vi "FocalMain.vi"() -> ()   [LabVIEW 2018]
uses:
  Clusters/FileDataChannel.ctl
  Clusters/WindSimMode.ctl
  Clusters/SimulationConstants.ctl
  Clusters/BladePitchMode.ctl
  Clusters/GenMode.ctl
  <vilib>/Platform/TimedLoop/XDataNode/timing_clust.ctl
  <vilib>/Platform/TimedLoop/XDataNode/nitl_modes.ctl
  <vilib>/Platform/TimedLoop/XDataNode/wakeup.ctl
  Clusters/IOSignals.ctl
  Clusters/RoscoParams.ctl
  Clusters/ArrayPairs.ctl
  Clusters/SwapArrayCluster.ctl
  Clusters/PitchCtrl.ctl
  Clusters/GenCtrl.ctl
  Clusters/ScalingEnum.ctl
  <vilib>/Utility/file.llb/Read Delimited Spreadsheet (DBL).vi
  SubVIs/InsertIntoArray_v2.vi
  <vilib>/platform/TimedLoop/XDataNode/XDataNode.xnode
  <vilib>/Platform/TimedLoop/XDataNode/XDNodeRunTimeDep.lvlib
  <resource>/objmgr/IndComECAT.rc
  <vilib>/ptbypt/NI_PtbyPt.lvlib
panel:
  out "error out":errorcluster
  in  "Torque Ctrl P-Gain":dbl=1.0
  in  "Pitch I-Gain":dbl
  out "Torque RAW (V)":dbl
  in  "Max Torque (MNm)":dbl=20.0
  in  "Velocity Ctrl I-Gain":dbl=0.5
  in  "Velocity Ctrl P-Gain":dbl=0.1
  in  "Torque Ctrl I-Gain":dbl=1.0
  out "Torque sine period MS (Nm) 2":dbl
  out "Torque sine amp MS (Nm)":dbl
  out "Torque setpoint (Nm)":dbl
  out "Torque Sensor (Nm)":dbl(knob) scale=-2.0..2.0
  in  "Torque sine period (s)":dbl=100.0
  in  "Torque sine amp (MNm)":dbl
  out "Motor Torque (Nm)":dbl(knob) scale=-2.0..2.0
  out "Torque sine mean MS (Nm)":dbl
  in  "Torque mean (MNm)":dbl
  out "Ramp time MS (s)":dbl
  out "Ramp target vel MS (rpm)":dbl
  out "Const. vel setpoint MS (rpm)":dbl
  in  "Ramp time (s)":dbl=100.0
  in  "Ramp target vel (rpm)":dbl=10.0
  in  "Const. vel setpoint (rpm)":dbl
  out "Sine period MS (s)":dbl
  out "Sine amp MS (deg)":dbl
  out "Sine Mean MS (deg)":dbl
  out "Const. setpoint MS (deg)":dbl
  in  "Generator operating mode":T1
  in  "Sine period (s)":dbl=100.0
  in  "Sine amp (deg)":dbl=15.0
  in  "Sine mean (deg)":dbl=1.0
  in  "Const. setpoint (deg)":dbl=10.0
  in  "Blade pitch operating mode":T2
  out "SIM-GenTorque_Nm":dbl
  in  "Wind Est. u(t=0)":dbl=5.0
  out "Wind Speed (m/s)":dbl
  out "Ramp time (s)":dbl
  in  "Ramp Time (s)":dbl=500.0
  in  "Ramp End u(m/s)":dbl=15.0
  in  "Ramp Start u(m/s)":dbl=5.0
  in  "Const. Amp (m/s)":dbl=5.0
  in  "Wind Simulation Mode":T3
  out "File Write (s)":dbl format="%5.1f"
  out "File Name":string
  out "State logic late?":bool
  out "Actual shaft Speed MS (rpm)":dbl(knob)=7.068579725455493e-05 scale=-100.0..100.0
  in  "Pitch P-Gain":dbl=12.0
  out "Axis 3 Fault":bool
  out "Axis 3 Warning":bool
  out "Axis 2 Fault":bool
  out "Axis 2 Warning":bool
  out "Axis 1 Fault":bool
  out "Axis 1 Warning":bool
  out "Axis 3 Operational":bool
  out "Axis 2 Operational":bool
  out "Axis 1 Operational":bool
  out "Pitch Axis 3":string
  out "Pitch Axis 2":string
  out "Pitch Axis 1":string
  in  "Clear Pitch Actuator Faults (x3)":bool
  in  "Enable Pitch Actuators (x3)":bool
  out "MS Pitch Blade 3 (deg)":dbl(knob) scale=0.0..30.0 scale format="%.2f"
  out "MS Pitch Blade 2 (deg)":dbl(knob) scale=0.0..30.0 scale format="%.2f"
  out "MS Pitch Blade 1 (deg)":dbl(knob) scale=0.0..30.0 scale format="%.2f"
  out "Generator Operational":bool
  in  "Clear Accelnet Faults":bool
  in  "Enable Accelnet":bool
  out "Generator Fault":bool
  out "Generator Warning":bool
  out "Main generator state":string
  out "Rosco Failed?":bool
  in  "Sine Freq (Hz)":dbl=0.009999999776482582
  in  "Sine Mean (m/s)":dbl=7.0
  in  "Sine Amp (m/s)":dbl
  out "Generator Torque (MNm)":dbl(knob) scale=0.0..35.0
  out "Generator Speed (rpm)":dbl(knob)=7.068579725455493e-05 scale=0.0..10.0
  in  "?":T4(tab)
  out "Generator Speed (ROSCO / SIM)":dynamicdata(graph)
  out "Torque (ROSCO/ SIM)":dynamicdata(graph)
  out "Pitch MS (ROSCO)":dynamicdata(graph)
  out "TSR":dynamicdata(graph)
  out "Generator Speed MS (Manual)":dynamicdata(graph)
  out "Pitch MS (Manual)":dynamicdata(graph)
  out "Torque MS (Manual)":dynamicdata(graph)
  out "Aero Torque":dynamicdata(graph)
  out "WindSpeed(m/s)":dbl(graph)
  in  "To VS_ControlMode":T5(ring)
  in  "Edit DISCON":bool
  out "DISCON.IN Contents":string
  in  "From VS_ControlMode":T5(ring)
  out "Rosco Return Message":string
  out "Setpoints":dbl[][](array[numeric])
  out "Pitch FS (deg)":dbl
  out "Time index":i32
  out "Time FS (s)":dbl
  out "Vel FS (rpm)":dbl
  out "Loop duration (ms)":i64
  out "Pitch axis 3 ctrl word":u16 format="%x"
  out "Pitch axis 2 ctrl word":u16 format="%x"
  out "avrSWAP":sgl[](array[numeric])
  out "OUT_DEBUG":dbl
  out "RT Loop Duration":i64
  out "Control Mode - Main Gen":u8
  out "WriteSDO Abort - Main Gen":u32
  out "ReadSDO Abort - Main Gen":u32
  out "Gen ctrl word":u16 format="%x"
  out "Pitch axis 1 ctrl word":u16 format="%x"
  out "Graphics Update t (s)":dbl format="%.1f"
  out "Effective rate (ms)":dbl format="%#.1f"
  out "WriteSDO Abort - Pitch 1":u32
  out "ReadSDO Abort - Pitch 1":u32
  out "Control Mode - Pitch 1":u8
  in  "Zero Pitch 1":bool
  in  "Zero Pitch 2":bool
  in  "Zero Pitch 3":bool
  out "SIM-Cp":dbl
  out "OUT_AEROTQ":dbl
  out "OUT_ROTSP":dbl
  out "SimulationConst":T6={"Ngear"=1.0, "RotorInertia"=318628128.0, "GeneratorEff"=0.9700000286102295, "RotorRadius"=120.0, "Rho"=1.225000023841858, "NumBlades"=1, "ScaleFactor"=3.0} {"RotorInertia" format="%.2f"}
  out "Scan Engine Mode":i32(ring)=2 items=["Initialization Mode", "Configuration Mode", "Active Mode", "Fault Mode"]
  out "Torque Setpoint (MNm)":dbl(knob) scale=0.0..35.0
  out "Pitch Setpoint (deg)":dbl(knob) scale=0.0..30.0 scale format="%.2f"
  out "Power (MW)":dbl(slide) scale=0.0..25.0 scale format="%.2f"
  out "SimLoop Late?":bool
  out "FIFO Loop Late?":bool
  in  "Base filename":string="rosco-tests"
  out "Writing":bool
  in  "WriteData":bool
  in  "?":T7
  out "#RT FIFO":u32
  in  "Stop LabVIEW":bool
  out "Time(s)":dbl format="%6.1f"
  out "RT Loop Late?":bool
  # "FOCAL Campaign 1"
  # "Processed quantities"
  # "FILEWRITING"
  # "MAIN GEN CONTROL"
  # "GENERATOR SIGNALS"
  # "PITCH ACTUATORS CONTROL"
  # "BLADE PITCH SIGNALS"
  # "ROSCO"
  # "WIND SPEED SIMULATOR"
  # "Axis 1"
  # "Axis 2"
  # "Axis 3"
  # "Operational"
  # "Warning"
  # "Error"
  # "Enter FS values"
  # "MS values"
  # "Enter FS values"
  # "MS values"
  # "TURBINE SPECIFICATIONS"
  # "RATED POWER: 15000000 W"
  # "RATED TORQUE: 19624046.66 Nm"
  # "RATED GEN SPEED: 0.79168 rad/s"
  # "ROSCO INPUTS"
  # "Pitch (deg)"
  # "Fan 1"
  # "Fan 20"
  # "Time"
  # "Vel (rpm)"
  # "Fan 10"
  # "Fan 30"
  # "SYSTEM"
  # "ROSCO"
  # "MAIN MOTOR"
  # "PITCH AXIS 1"
  # "PITCH AXIS 2"
  # "PITCH AXIS 3"
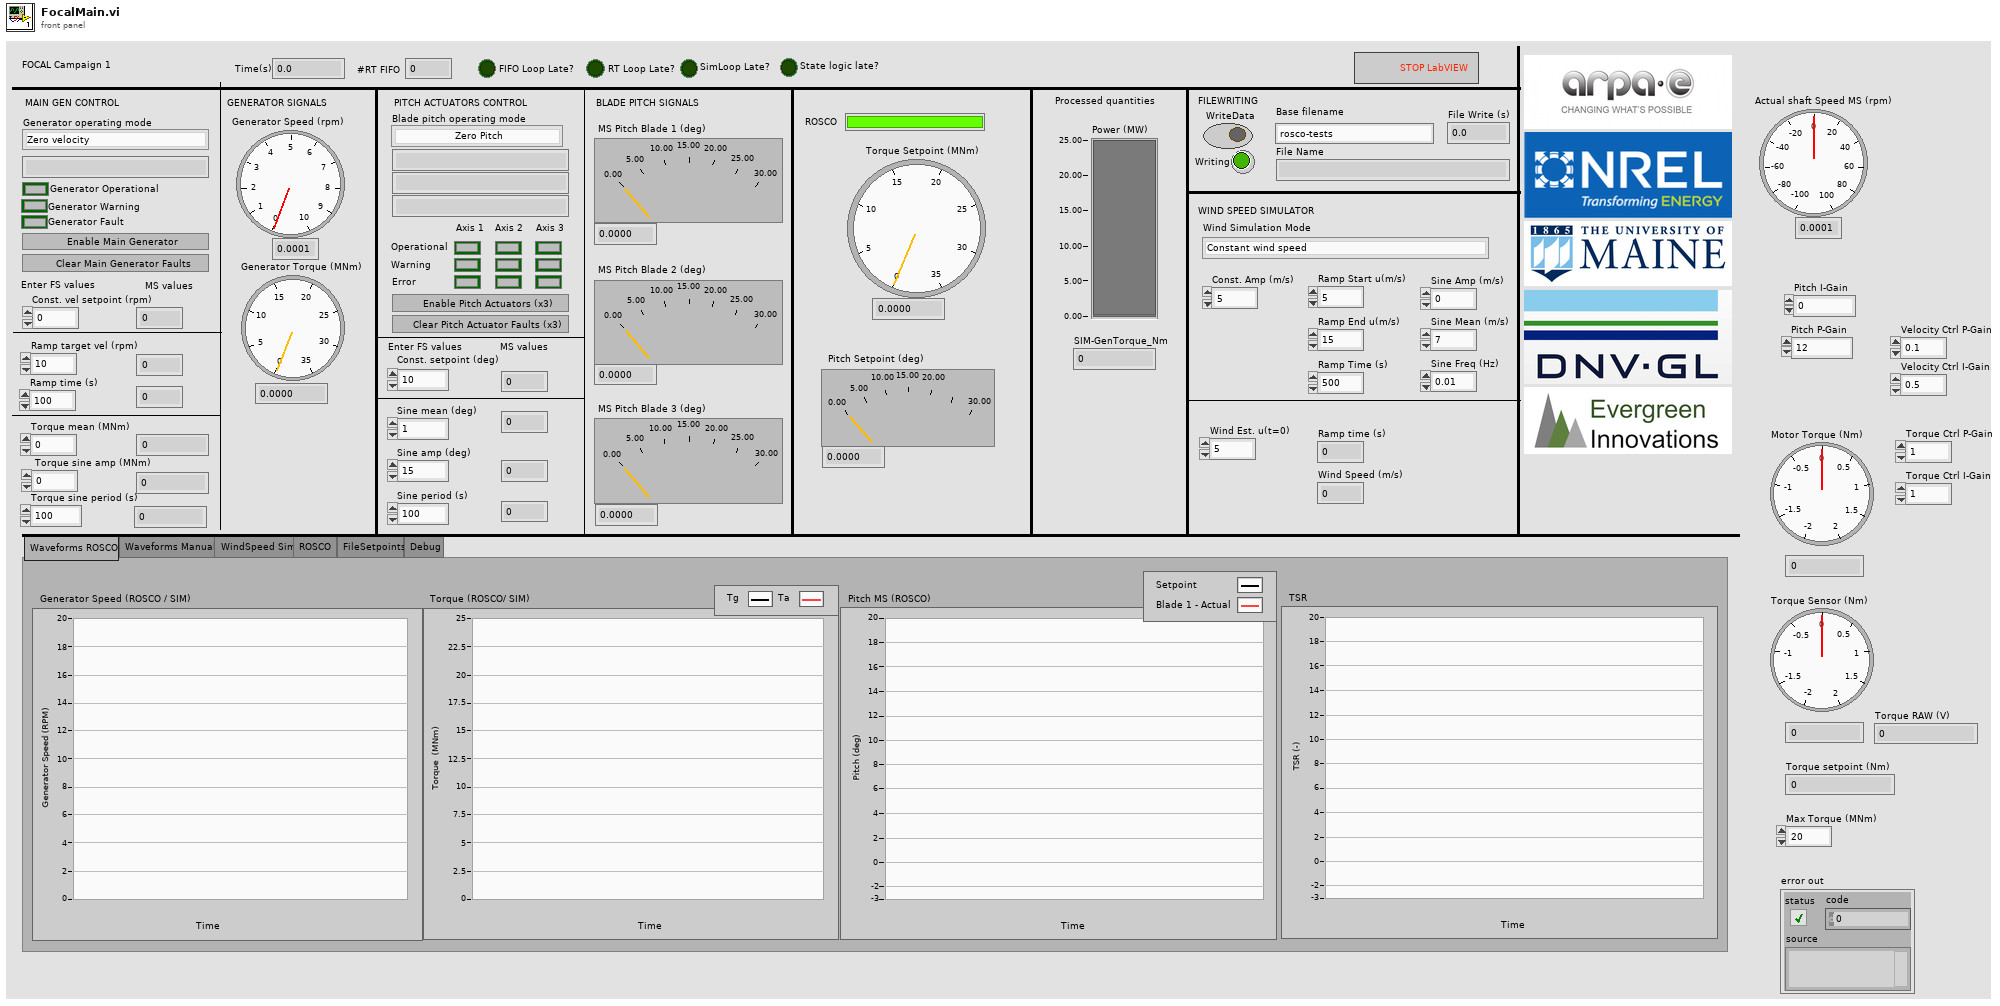
[diagram p1: front panel]
types:
  T1 = typedef "GenMode.ctl" = enum16{"Zero velocity", "Velocity from File", "Constant velocity", "Ramped Velocity", "Sine Torque", "ROSCO"}
  T2 = typedef "BladePitchMode.ctl" = enum16{"Zero Pitch", "Pitch from File", "Constant pitch angle", "Harmonic pitch angle", "ROSCO controlled"}
  T3 = typedef "WindSimMode.ctl" = enum16{"Constant wind speed", "Ramped wind speed", "Sine wind speed"}
  T4 = enum32{"Waveforms ROSCO", "Waveforms Manual", "WindSpeed Sim", "ROSCO", "FileSetpoints", "Debug"}
  T5 = enum16{"Constant Torque", "Constant Power", "PI Control"}
  T6 = typedef "SimulationConstants.ctl" = cluster{"Ngear":dbl, "RotorInertia":dbl, "GeneratorEff":dbl, "RotorRadius":sgl, "Rho":dbl, "NumBlades":i32, "ScaleFactor":dbl}
  T7 = typedef "FileDataChannel.ctl" = cluster{"genSpeed_rad_s":dbl, "genTorque_Nm":dbl, "dataLoopCounter":dbl, "genStatus":dbl, "pitch1Position_rad":dbl, "pitch1Velocity_rad_s":dbl, "pitch1Status":dbl, "dataTime_s":dbl, "genPosition_rad":dbl, "pitch2Position_rad":dbl, "pitch2Velocity_rad_s":dbl, "pitch2Status":dbl, "pitch3Position_rad":dbl, "pitch3Velocity_rad_s":dbl, "pitch3Status":dbl, "pitchSetpoint_rad":dbl, "torqueSetpoint_Nm":dbl, "simUWind_m_s":dbl, "simGenSpeed_rad_s":dbl, "simTa_Nm":dbl, "simCp":dbl}
  T8 = typedef "IOSignals.ctl" = cluster{"mainGenPosition (rad)":dbl, "mainGenTorque (Nm)":dbl, "mainGenVelocity (rad/s)":dbl, "mainGenStatus":u16, "pitch1Position (rad)":dbl, "pitch1Velocity (rad/s)":dbl, "pitch1Status":u16, "pitch2Position (rad)":dbl, "pitch2Velocity (rad/s)":dbl, "pitch2Status":u16, "pitch3Position (rad)":dbl, "pitch3Velocity (rad/s)":dbl, "pitch3Status":u16, "pitch1PosOfst (rad)":dbl, "pitch2PosOfst (rad)":dbl, "pitch3PosOfst (rad)":dbl, "torqueSensor (Nm)":dbl}
  T9 = typedef "RoscoParams.ctl" = cluster{"avrSWAP":sgl[], "aviFAIL":i32, "avcMSG":string, "ReturnValue":i32}
  T10 = typedef "ArrayPairs.ctl" = cluster{"iStatus":T11, "TIME":T11, "DT":T11, "Blade1PitchPos_rad":T11, "VS_MECHGENPWR":T11, "VS_GENPWR":T11, "GEN_SPEED":T11, "ROTOR_SPEED":T11, "GENTQMEAS":T11, "Y_M":T11, "HORWINDV":T11, "ROOTMOOP1":T11, "ROOTMOOP2":T11, "Blade2PitchPos_rad":T11, "Blade3PitchPos_rad":T11, "ROOTMOOP3":T11, "AVCMSG_SIZE":T11, "INFILE_SIZE ":T11, "OUTFILE_SIZE ":T11, "FA_ACC":T11, "NUM_BLADES":T11, "BladePitchSetpoint_rad":T11, "TorqueSetpoint_Nm":T11, "OUT_AEROTQ":T11, "Out.RotSpeed ":T11, "Out.DEBUG":T11}
  T11 = typedef "SwapArrayCluster.ctl" = cluster{"Index":i32, "Value":dbl}
  T12 = typedef "XDNodeRunTimeDep.lvlib/timing_clust.ctl" = cluster{"Expected End [f-1]":u64, "Actual End [f-1]":u64, "Finished Late? [f-1]":bool, "Expected End [i-1]":u64, "Actual End [i-1]":u64, "Finished Late? [i-1]":bool, "Expected Start [i]":u64, "Actual Start [i]":u64, "Expected Start [f]":u64, "Actual Start [f]":u64, "Source Name":string, "Structure Name":string, "Period":i64, "Deadline":i64, "Offset":i64, "Start":i64, "Priority":i32, "Timeout":i32, "Mode":T13, "Wakeup Reason":T14, "Error":errorcluster, "Source Type":string, "Secondary Source Type":string, "Global End Time":u64, "Global Start Time":u64, "Frame Duration":u64, "Iteration Duration":u64, "Assigned CPU":i32, "I/O Scan Engine Mode":u32}
  T13 = typedef "XDNodeRunTimeDep.lvlib/nitl_modes.ctl" = enum32{"No Change", "Process missed periods, maintain original phase", "Discard missed periods, maintain original phase", "Process missed periods, ignore original phase", "Discard missed periods, ignore original phase"}
  T14 = typedef "XDNodeRunTimeDep.lvlib/wakeup.ctl" = enum32{"Normal", "Aborted", "Asynchronous wakeup", "Timing source error", "Timed loop error", "Timeout"}
  T15 = typedef "PitchCtrl.ctl" = cluster{"P-Gain":dbl, "Blade pitch operating mode":T2, "Constant setpoint (deg)":dbl, "Sine mean (deg)":dbl, "Sine amp (deg)":dbl, "Sine period (s)":dbl, "I-Gain":dbl, "Axis 1 On":bool, "Axis 2 On":bool, "Axis 3 On":bool, "Pitch from File (deg)":dbl}
  T16 = typedef "GenCtrl.ctl" = cluster{"Generator operating mode":T1, "Constant velocity setpoint (rpm)":dbl, "Ramp target velocity (rpm)":dbl, "Ramp time (s)":dbl, "Sine mean (Nm)":dbl, "Sine amp (Nm)":dbl, "Sine period (s)":dbl, "Torque Ctrl I-Gain":dbl, "Velocity Ctrl P-Gain":dbl, "Velocity Ctrl I-Gain":dbl, "Max Torque (Nm)":dbl, "GeneratorOn":bool, "Torque Ctrl P-Gain":dbl, "From file velocity (rpm)":dbl}
  T17 = typedef "ScalingEnum.ctl" = enum16{"Model scale -> Full scale", "Full scale -> Model scale"}
  T18 = typedef "ElmoState.ctl" = cluster{"Elmo State":string, "Elmo Operational":bool, "Elmo Warning":bool, "Elmo Fault":bool}
  T19 = typedef "AccelnetState.ctl" = cluster{"State String":string, "Accelnet Warning":bool, "Accelnet Fault":bool, "Accelnet Operational":bool}
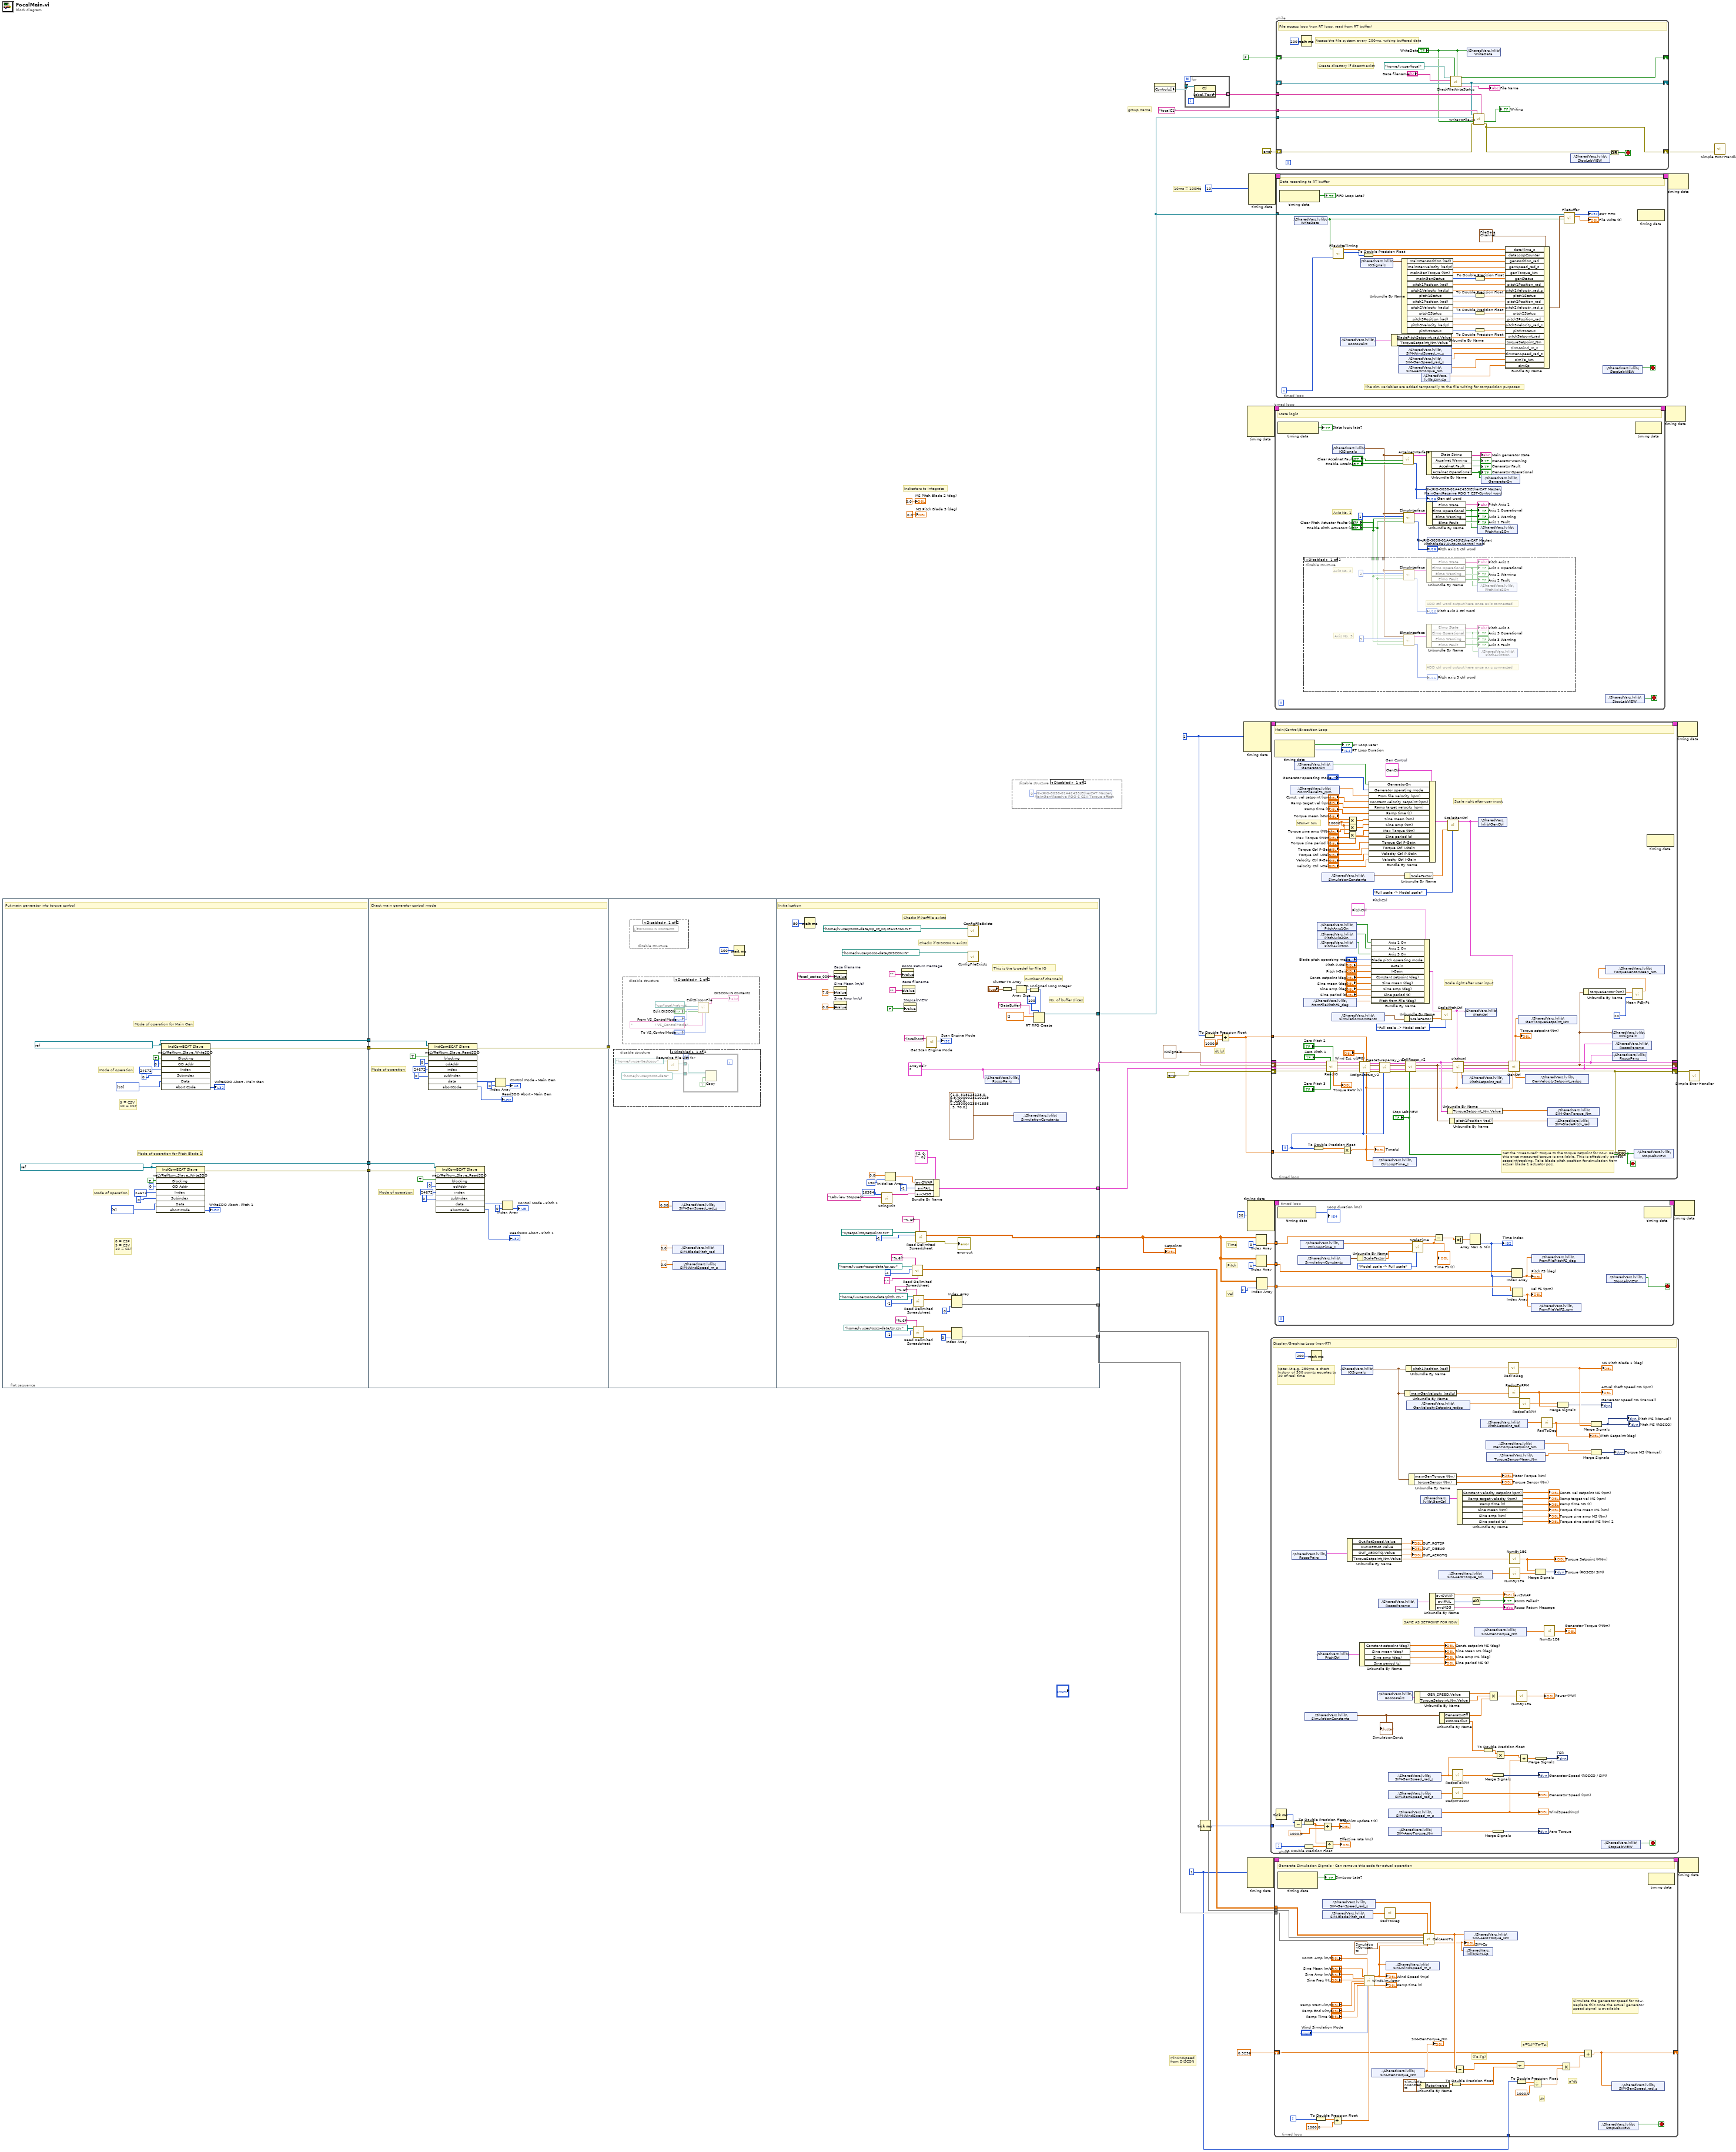
[diagram p0: block diagram]
diagram:
  w16 = i64 2 ("Period")
  w23 = i64 1 ("Period")
  # "Vel"
  # "Pitch"
  # "Time"
  # "MinOMSpeed\nfrom DISCON"
  # "dt (s)"
  # "10ms = 100Hz"
  # "group name"
  # "Indicators to integrate"
  n1 = flat-sequence {
    tunnel: [w57] -> w33
    tunnel: [w58] -> w32
    tunnel: [w50] -> w25
    tunnel: [w49] -> w24
    tunnel: w33 -> [w77]
    tunnel: w32 -> [w76]
    tunnel: [w75] -> w31
    tunnel: w25 -> [w66]
    tunnel: w24 -> [w65]
    tunnel: w31 -> [_]
    tunnel: [w146] -> w27
    tunnel: [w139] -> w40
    tunnel: [w125] -> w39
    tunnel: [w128] -> w38
    tunnel: [w127] -> w37
    tunnel: [w110] -> w36
    tunnel: [w103] -> w4
    frame #0 {
      w50 = refnum<k21> "ni.var.io://ni-crio-9038-01a42455/EtherCAT Master/PitchBlade1" ("Slave Constant")
      w57 = refnum<k21> "ni.var.io://ni-crio-9038-01a42455/EtherCAT Master/MainGen" ("Slave Constant")
      # "Mode of operation for Pitch Blade 1"
      # "Mode of operation for Main Gen"
      # "Mode of operation"
      # "8 = CSP \n9 = CSV\n10 = CST"
      # "Mode of operation"
      # "9 = CSV\n10 = CST"
      # "Put main generator into torque control"
      n2 = invoke class="IndComECAT Slave" method="neLVRefNum_Slave_WriteSDO"(reference=w50, "Blocking"=TRUE, "OD Addr"=u16 0, "Index"=u16 24672, "Subindex"=u8 0, "Data"=u8[] [9]) -> (error out=w49:errorcluster, "Abort Code"=→"WriteSDO Abort - Pitch 1":u32)  [unwired: 3 in, 7 out]
      n3 = invoke class="IndComECAT Slave" method="neLVRefNum_Slave_WriteSDO"(reference=w57, "Blocking"=TRUE, "OD Addr"=u16 0, "Index"=u16 24672, "Subindex"=u8 0, "Data"=u8[] [10]) -> (error out=w58:errorcluster, "Abort Code"=→"WriteSDO Abort - Main Gen":u32)  [unwired: 3 in, 7 out]
    }
    frame #1 {
      # "Mode of operation"
      # "Mode of operation"
      # "Check main generator control mode"
      n4 = invoke class="IndComECAT Slave" method="neLVRefNum_Slave_ReadSDO"(reference=w77, error in=w76, "blocking"=TRUE, "odAddr"=u16 0 ("OD address"), "index"=u16 24672 ("Index"), "subIndex"=u8 0 ("Subindex")) -> (error out=w75:errorcluster, "data"=w80:u8[], "abortCode"=→"ReadSDO Abort - Main Gen":u32)  [unwired: 3 in, 6 out]
      n5 = invoke class="IndComECAT Slave" method="neLVRefNum_Slave_ReadSDO"(reference=w66, error in=w65, "blocking"=TRUE, "odAddr"=u16 0 ("OD address"), "index"=u16 24672 ("Index"), "subIndex"=u8 0 ("Subindex")) -> ("data"=w69:u8[], "abortCode"=→"ReadSDO Abort - Pitch 1":u32)  [unwired: 3 in, 7 out]
      n6 = Index Array(array=w80, index=0) -> (element=→"Control Mode - Main Gen":u8)
      n7 = Index Array(array=w69, index=0) -> (element=→"Control Mode - Pitch 1":u8)
    }
    frame #2 {
      n8 = disable-structure shown="Disabled" {
        frame Disabled {
          n9 = call <vilib>:"Recursive File List.vi"("Folder Path"=path "/home/lvuser/testcopy" ("path")) -> ("All Files in Dir"=w91:path[])  [unwired: 6 in, 4 out]
          n10 = for {
            tunnel: path "/home/lvuser/rosco-data" ("target path (use dialog)") -> [w95]
            tunnel: w91 -> [w94] mode=indexing
            n11 = Copy(9:TRUE ("overwrite (F)"), 10:w95, 11:w94) -> ()  [unwired: 2 in, 3 out]
          }
        }
        frame Enabled {
        }
      }
      n12 = disable-structure shown="Disabled" {
        frame Disabled {
          n13 = call "EditDisconFile.vi"("To VS_ControlMode"="To VS_ControlMode", "Append"="                   ! VS_ControlMode", "Edit DISCON"="Edit DISCON", "From VS_ControlMode"="From VS_ControlMode", "path"=path "/usr/local/natinst/labview/DISCON.IN") -> ("data"=→"DISCON.IN Contents":string)  [unwired: 4 in, 1 out]
        }
        frame Enabled {
        }
      }
      n14 = disable-structure shown="Disabled" {
        frame Disabled {
          n15 = local read "DISCON.IN Contents"() -> ()  [unwired: 1 in]
        }
        frame Enabled {
        }
      }
      n16 = shared-variable ".\\SharedVars.lvlib\\SIM-GenSpeed_rad_s"(0.009999999776482582 ("RotorSpeed(rad/s)")) -> ()  [unwired: 1 in, 1 out]
      n17 = shared-variable ".\\SharedVars.lvlib\\SIM-BladePitch_rad"(0.0 ("ecat-BladePitch")) -> ()  [unwired: 1 in, 1 out]
      n18 = shared-variable ".\\SharedVars.lvlib\\SIM-WindSpeed_m_s"(0.0 ("WindSpeedSim")) -> ()  [unwired: 1 in, 1 out]
      n19 = Wait (ms)(milliseconds to wait=u32 100) -> ()  [unwired: 1 out]
    }
    frame #3 {
      w110 = T10 {"iStatus"={"Index"=0, "Value"=0.0}, "TIME"={"Index"=1, "Value"=0.0}, "DT"={"Index"=2, "Value"=0.0}, "Blade1PitchPos_rad"={"Index"=3, "Value"=0.0}, "VS_MECHGENPWR"={"Index"=13, "Value"=0.0}, "VS_GENPWR"={"Index"=14, "Value"=0.0}, "GEN_SPEED"={"Index"=19, "Value"=0.0}, "ROTOR_SPEED"={"Index"=20, "Value"=0.0}, "GENTQMEAS"={"Index"=22, "Value"=0.0}, "Y_M"={"Index"=23, "Value"=0.0}, "HORWINDV"={"Index"=26, "Value"=0.0}, "ROOTMOOP1"={"Index"=29, "Value"=0.0}, "ROOTMOOP2"={"Index"=30, "Value"=0.0}, "Blade2PitchPos_rad"={"Index"=32, "Value"=0.0}, "Blade3PitchPos_rad"={"Index"=33, "Value"=0.0}, "ROOTMOOP3"={"Index"=31, "Value"=0.0}, "AVCMSG_SIZE"={"Index"=48, "Value"=0.0}, "INFILE_SIZE "={"Index"=49, "Value"=0.0}, "OUTFILE_SIZE "={"Index"=50, "Value"=0.0}, "FA_ACC"={"Index"=52, "Value"=0.0}, "NUM_BLADES"={"Index"=60, "Value"=0.0}, "BladePitchSetpoint_rad"={"Index"=44, "Value"=0.0}, "TorqueSetpoint_Nm"={"Index"=46, "Value"=0.0}, "OUT_AEROTQ"={"Index"=91, "Value"=0.0}, "Out.RotSpeed "={"Index"=92, "Value"=0.0}, "Out.DEBUG"={"Index"=93, "Value"=0.0}} ("ArrayPairs")
      # "No. of buffer slices"
      # "This is the typedef for File IO"
      # "number of channels"
      # "Checks if PerfFile exists"
      # "Checks if DISCON.IN exists"
      # "Initialization"
      n20 = Wait (ms)(milliseconds to wait=u32 50) -> ()  [unwired: 1 out]
      n21 = property on="Base filename" class="Str"("Value"="focal_series_000" ("Base filename")) -> ()  [unwired: 2 in, 2 out]
      n22 = property on="Sine Mean (m/s)" class="DigNum (strict)"("Value"=7.0 ("GenSpeed Mean")) -> ()  [unwired: 2 in, 2 out]
      n23 = property on="Sine Amp (m/s)" class="DigNum (strict)"("Value"=0.0 ("GenSpeeed Amplitude")) -> ()  [unwired: 2 in, 2 out]
      n24 = call "StringInit.vi"("accOUTNAME"="Labview Stopped", "dimension size"=16384) -> ("result string"=w111:string)  [unwired: 9 in]
      n25 = Initialize Array(sgl 0.0 ("element"), 150 ("dimension size")) -> (w118:sgl[])
      n26 = property on="Rosco Return Message" class="Str"("Value"="") -> ()  [unwired: 2 in, 2 out]
      n27 = property on="Base filename" class="Str"("Value"="") -> ()  [unwired: 2 in, 2 out]
      n28 = property on="StopLabVIEW" class="Bool (strict)"("Value"=FALSE) -> ()  [unwired: 2 in, 2 out]
      n29 = call-poly <vilib>:"Read Delimited Spreadsheet.vi"("file path (dialog if empty)"=path "/home/lvuser/rosco-data/cp.csv", "format (%.3f)"="%.6f", "number of rows (all:-1)"=-1, "delimiter (\\t)"="," ("delimiter (\\t)")) -> ("all rows"=w125:dbl[][])  [unwired: 6 in, 5 out]
      n30 = call-poly <vilib>:"Read Delimited Spreadsheet.vi"("file path (dialog if empty)"=path "/home/lvuser/rosco-data/pitch.csv", "format (%.3f)"="%.6f", "number of rows (all:-1)"=-1) -> ("all rows"=w132:dbl[][])  [unwired: 7 in, 5 out]
      n31 = call-poly <vilib>:"Read Delimited Spreadsheet.vi"("file path (dialog if empty)"=path "/home/lvuser/rosco-data/tsr.csv", "format (%.3f)"="%.6f", "number of rows (all:-1)"=-1) -> ("all rows"=w134:dbl[][])  [unwired: 7 in, 5 out]
      n32 = Bundle By Name(cluster=T9 {"avrSWAP"=[], "aviFAIL"=0, "avcMSG"="", "ReturnValue"=0}, "avrSWAP"=w118, "aviFAIL"=-1, "avcMSG"=w111) -> (w139:T9)
      n33 = call-poly <vilib>:"Read Delimited Spreadsheet.vi"("file path (dialog if empty)"=path "C:/setpoints/setpoints.txt", "format (%.3f)"="%.6f", "number of rows (all:-1)"=-1) -> ("all rows"=w103:dbl[][], "error out"=→"error out":errorcluster)  [unwired: 7 in, 4 out]
      n34 = call <vilib>:"Get Scan Engine Mode.vi"("target address (localhost)"="localhost") -> ("mode"=→"Scan Engine Mode":i32)  [unwired: 9 in, 1 out]
      n35 = Index Array(array=w132, index (col)=0 ("disabled index (col)")) -> (element=w128:dbl[])  [unwired: 1 in]
      n36 = Index Array(array=w134, index (col)=0 ("disabled index (col)")) -> (element=w127:dbl[])  [unwired: 1 in]
      n37 = call "ConfigFileExists.vi"("path"=path "/home/lvuser/rosco-data/Cp_Ct_Cq.IEA15MW.txt") -> ()  [unwired: 11 in]
      n38 = call "ConfigFileExists.vi"("path"=path "/home/lvuser/rosco-data/DISCON.IN") -> ()  [unwired: 11 in]
      n39 = shared-variable ".\\SharedVars.lvlib\\RoscoPairs"(w110) -> ()  [unwired: 1 in, 1 out]
      n40 = Cluster To Array(cluster="?") -> (array=w114:dbl[])
      n41 = shared-variable ".\\SharedVars.lvlib\\SimulationConstants"(T6 {"Ngear"=1.0, "RotorInertia"=318628128.0, "GeneratorEff"=0.9700000286102295, "RotorRadius"=120.0, "Rho"=1.225000023841858, "NumBlades"=3, "ScaleFactor"=70.0} ("SimulationConst")) -> ()  [unwired: 1 in, 1 out]
      n42 = Array Size(array=w114) -> (size(s)=w113:i32)
      n43 = To Unsigned Long Integer(number=w113) -> (unsigned 32bit integer=w112:u32)
      n44 = RT FIFO Create(0:"DataBuffer" ("name (unnamed)"), 1:dbl[] [] ("appended array"), 4:u32 100, 6:w112) -> (8:w146:refnum<k33>)  [unwired: 4 in, 2 out]
    }
  }
  n45 = disable-structure shown="Disabled" {
    frame Disabled {
      n46 = shared-variable "NI-cRIO-9038-01A42455\\EtherCAT Master\\MainGen\\Receive PDO 6 CSV-Torque offset"(i16 0 ("Receive PDO 6 CSV-Torque offset")) -> ()  [unwired: 1 in, 1 out]
    }
    frame Enabled {
    }
  }
  n47 = property class="Clust (strict)"() -> ("Controls[]"=w46:refnum<vi>[])  [unwired: 2 in, 2 out]
  n48 = for {
    tunnel: w46 -> [w156] mode=indexing
    tunnel: [w155] -> w45 mode=indexing
    n49 = property class="Ctl"(reference=w156) -> ("Label.Text"=w155:string)  [unwired: 1 in, 2 out]
  }
  n50 = Tick Count (ms)() -> (millisecond timer value=w26:u32)
  n51 = To Double Precision Float(number=w16) -> (double precision float=w15:dbl)
  n52 = Divide(x=w15, y=1000.0) -> (x/y=w14:dbl)
  n53 = node-c288(w16) -> (w22:T12)  [unwired: 3 in]
  n54 = node-c288(w23) -> (w48:T12)  [unwired: 3 in]
  n55 = node-c288() -> (w35:T12)  [unwired: 4 in]
  n56 = node-c288(i64 50 ("Period")) -> (w10:T12)  [unwired: 3 in]
  n57 = node-c288(i64 10 ("Period")) -> (w30:T12)  [unwired: 3 in]
  n58 = Index Array(array=w4, index (col)=0 ("disabled index (col)")) -> (element=w2:dbl[])  [unwired: 1 in]
  n59 = Index Array(array=w4, index (col)=1 ("disabled index (col)")) -> (element=w3:dbl[])  [unwired: 1 in]
  n60 = Index Array(array=w4, index (col)=2 ("disabled index (col)")) -> (element=w1:dbl[])  [unwired: 1 in]
  n61 = while {
    tunnel: w26 -> [w199]
    i -> [w193]
    stop <- w231 stop-if-true
    # "SAME AS SETPOINT FOR NOW"
    # "Note: At e.g. 250ms, a chart history of 500 points equates to 20 of real time"
    # "Display/Graphics Loop (non-RT)"
    n62 = Tick Count (ms)() -> (millisecond timer value=w200:u32)
    n63 = shared-variable ".\\SharedVars.lvlib\\RoscoPairs"() -> (w214:T10)  [unwired: 1 in, 1 out]
    n64 = Subtract(x=w200, y=w199) -> (x-y=w196:u32)
    n65 = To Double Precision Float(number=w193) -> (double precision float=w194:dbl)
    n66 = To Double Precision Float(number=w196) -> (double precision float=w195:dbl)
    n67 = shared-variable ".\\SharedVars.lvlib\\SimulationConstants"() -> (w183:T6)  [unwired: 1 in, 1 out]
    "SimulationConst" <- w183
    n68 = Wait (ms)(milliseconds to wait=u32 200 ("Period")) -> ()  [unwired: 1 out]
    n69 = shared-variable ".\\SharedVars.lvlib\\PitchCtrl"() -> (w188:T15)  [unwired: 1 in, 1 out]
    n70 = Divide(x=w195, y=1000.0) -> (x/y=→"Graphics Update t (s)":dbl)
    n71 = Divide(x=w195, y=w194) -> (x/y=→"Effective rate (ms)":dbl)
    n72 = shared-variable ".\\SharedVars.lvlib\\IOSignals"() -> (w167:T8)  [unwired: 1 in, 1 out]
    n73 = Unbundle By Name(w214) -> ("Out.RotSpeed.Value"=→"OUT_ROTSP":dbl, "Out.DEBUG.Value"=→"OUT_DEBUG":dbl, "OUT_AEROTQ.Value"=→"OUT_AEROTQ":dbl, "TorqueSetpoint_Nm.Value"=w213:dbl)
    n74 = Unbundle By Name(w188) -> ("Constant setpoint (deg)"=→"Const. setpoint MS (deg)":dbl, "Sine mean (deg)"=→"Sine Mean MS (deg)":dbl, "Sine amp (deg)"=→"Sine amp MS (deg)":dbl, "Sine period (s)"=→"Sine period MS (s)":dbl)
    n75 = shared-variable ".\\SharedVars.lvlib\\RoscoPairs"() -> (w211:T10)  [unwired: 1 in, 1 out]
    n76 = shared-variable ".\\SharedVars.lvlib\\RoscoParams"() -> (w230:T9)  [unwired: 1 in, 1 out]
    n77 = shared-variable ".\\SharedVars.lvlib\\SIM-GenSpeed_rad_s"() -> (w175:dbl)  [unwired: 1 in, 1 out]
    n78 = shared-variable ".\\SharedVars.lvlib\\SIM-GenSpeed_rad_s"() -> (w207:dbl)  [unwired: 1 in, 1 out]
    n79 = shared-variable ".\\SharedVars.lvlib\\SIM-WindSpeed_m_s"() -> (w171:dbl)  [unwired: 1 in, 1 out]
    "WindSpeed(m/s)" <- w171
    n80 = shared-variable ".\\SharedVars.lvlib\\SIM-AeroTorque_Nm"() -> (w224:dbl)  [unwired: 1 in, 1 out]
    n81 = Unbundle By Name(w167) -> ("mainGenVelocity (rad/s)"=w161:dbl)
    n82 = Unbundle By Name(w167) -> ("pitch1Position (rad)"=w191:dbl)
    n83 = shared-variable ".\\SharedVars.lvlib\\GenVelocitySetpoint_radps"() -> (w163:dbl)  [unwired: 1 in, 1 out]
    n84 = Unbundle By Name(w167) -> ("mainGenTorque (Nm)"=→"Motor Torque (Nm)":dbl, "torqueSensor (Nm)"=→"Torque Sensor (Nm)":dbl)
    n85 = Unbundle By Name(w211) -> ("GEN_SPEED.Value"=w210:dbl, "TorqueSetpoint_Nm.Value"=w209:dbl)
    n86 = shared-variable ".\\SharedVars.lvlib\\GenCtrl"() -> (w182:T16)  [unwired: 1 in, 1 out]
    n87 = Unbundle By Name(w230) -> ("avrSWAP"=→"avrSWAP":sgl[], "aviFAIL"=w228:i32, "avcMSG"=→"Rosco Return Message":string)
    n88 = shared-variable ".\\SharedVars.lvlib\\SIM-AeroTorque_Nm"() -> (w220:dbl)  [unwired: 1 in, 1 out]
    n89 = Unbundle By Name(w183) -> ("GeneratorEff"=w212:dbl, "RotorRadius"=w174:sgl)
    n90 = call "RadpsToRPM.vi"("radps"=w175) -> ("rpm"=w205:dbl)
    n91 = call "RadpsToRPM.vi"("radps"=w207) -> ("rpm"=→"Generator Speed (rpm)":dbl)
    n92 = Unbundle By Name(w182) -> ("Constant velocity setpoint (rpm)"=→"Const. vel setpoint MS (rpm)":dbl, "Ramp target velocity (rpm)"=→"Ramp target vel MS (rpm)":dbl, "Ramp time (s)"=→"Ramp time MS (s)":dbl, "Sine mean (Nm)"=→"Torque sine mean MS (Nm)":dbl, "Sine amp (Nm)"=→"Torque sine amp MS (Nm)":dbl, "Sine period (s)"=→"Torque sine period MS (Nm) 2":dbl)
    n93 = Not Equal To 0?(x=w228) -> (x != 0?=→"Rosco Failed?":bool)
    n94 = shared-variable ".\\SharedVars.lvlib\\SIM-GenTorque_Nm"() -> (w203:dbl)  [unwired: 1 in, 1 out]
    n95 = shared-variable ".\\SharedVars.lvlib\\PitchSetpoint_rad"() -> (w189:dbl)  [unwired: 1 in, 1 out]
    n96 = To Double Precision Float(number=w174) -> (double precision float=w173:dbl)
    n97 = shared-variable ".\\SharedVars.lvlib\\GenTorqueSetpoint_Nm"() -> (w158:dbl)  [unwired: 1 in, 1 out]
    n98 = shared-variable ".\\SharedVars.lvlib\\TorqueSensorMean_Nm"() -> (w157:dbl)  [unwired: 1 in, 1 out]
    n99 = Compound Arithmetic op=MULTIPLY(w210, w209, w212) -> (w208:dbl)
    n100 = Merge Signals(w205) -> (→"Generator Speed (ROSCO / SIM)":dynamicdata)
    n101 = Merge Signals(w224) -> (→"Aero Torque":dynamicdata)
    n102 = Multiply(x=w173, y=w175) -> (x*y=w172:dbl)
    n103 = call "RadToDeg.vi"("rad"=w191) -> ("deg"=w190:dbl)
    "MS Pitch Blade 1 (deg)" <- w190
    n104 = call "RadpsToRPM.vi"("radps"=w161) -> ("rpm"=w177:dbl)
    "Actual shaft Speed MS (rpm)" <- w177
    n105 = call "NumBy1E6.vi"("x"=w213) -> ("Mx"=w221:dbl)
    "Torque Setpoint (MNm)" <- w221
    n106 = call "NumBy1E6.vi"("x"=w220) -> ("Mx"=w219:dbl)
    n107 = call "NumBy1E6.vi"("x"=w208) -> ("Mx"=→"Power (MW)":dbl)
    n108 = Divide(x=w172, y=w171) -> (x/y=w170:dbl)
    n109 = call "RadpsToRPM.vi"("radps"=w163) -> ("rpm"=w162:dbl)
    n110 = Merge Signals(w221, w219) -> (→"Torque (ROSCO/ SIM)":dynamicdata)
    n111 = Merge Signals(w170) -> (→"TSR":dynamicdata)
    n112 = call "RadToDeg.vi"("rad"=w189) -> ("deg"=w204:dbl)
    "Pitch Setpoint (deg)" <- w204
    n113 = call "NumBy1E6.vi"("x"=w203) -> ("Mx"=→"Generator Torque (MNm)":dbl)
    n114 = Merge Signals(w162, w177) -> (→"Generator Speed MS (Manual)":dynamicdata)
    n115 = Merge Signals(w158, w157) -> (→"Torque MS (Manual)":dynamicdata)
    n116 = Merge Signals(w204, w190) -> (→"Pitch MS (ROSCO)" →"Pitch MS (Manual)":dynamicdata)
    n117 = shared-variable ".\\SharedVars.lvlib\\StopLabVIEW"() -> (w231:bool)  [unwired: 1 in, 1 out]
  }
  n118 = timed-loop {
    timing: w22 -> [_]
    timing-out: [_] -> w21
    shift-right: [w264] -> _
    shift-left: w40 -> [w316]
    shift-right: [w263] -> w19
    shift-left: errorcluster {"status"=FALSE, "code"=0, "source"=""} ("error out") -> [w315]
    shift-right: [w265] -> _
    shift-left: w36 -> [w317]
    shift-right: [w240] -> _
    shift-left: T8 {"mainGenPosition (rad)"=0.0, "mainGenTorque (Nm)"=0.0, "mainGenVelocity (rad/s)"=0.0, "mainGenStatus"=0, "pitch1Position (rad)"=0.0, "pitch1Velocity (rad/s)"=0.0, "pitch1Status"=0, "pitch2Position (rad)"=0.0, "pitch2Velocity (rad/s)"=0.0, "pitch2Status"=0, "pitch3Position (rad)"=0.0, "pitch3Velocity (rad/s)"=0.0, "pitch3Status"=0, "pitch1PosOfst (rad)"=0.0, "pitch2PosOfst (rad)"=0.0, "pitch3PosOfst (rad)"=0.0, "torqueSensor (Nm)"=0.0} -> [w314]
    tunnel: w14 -> [w309]
    tunnel: w14 -> [w308]
    i -> [w289]
    stop <- w321 stop-if-true
    w258 = 1000000.0 ("y")
    w277 = T16 {"Generator operating mode"=enum."Zero velocity", "Constant velocity setpoint (rpm)"=0.0, "Ramp target velocity (rpm)"=0.0, "Ramp time (s)"=0.0, "Sine mean (Nm)"=0.0, "Sine amp (Nm)"=0.0, "Sine period (s)"=0.0, "Torque Ctrl I-Gain"=0.0, "Velocity Ctrl P-Gain"=0.0, "Velocity Ctrl I-Gain"=0.0, "Max Torque (Nm)"=0.0, "GeneratorOn"=FALSE, "Torque Ctrl P-Gain"=0.0, "From file velocity (rpm)"=0.0}  # Gen Control
    w284 = T15 {"P-Gain"=0.0, "Blade pitch operating mode"=enum."Constant pitch angle", "Constant setpoint (deg)"=0.0, "Sine mean (deg)"=0.0, "Sine amp (deg)"=0.0, "Sine period (s)"=0.0, "I-Gain"=0.0, "Axis 1 On"=FALSE, "Axis 2 On"=FALSE, "Axis 3 On"=FALSE, "Pitch from File (deg)"=0.0}  # PitchCtrl
    # "MNm-> Nm"
    # "Scale right after user input"
    # "Scale right after user input"
    # "Set the \"measured\" torque to the torque setpoint for now. Remove this once measured torque is available. This is effectively perfect setpoint tracking. Take blade pitch position for simulation from actual blade 1 actuator pos."
    # "Main/Control/Execution Loop"
    n119 = node-c288() -> (→"RT Loop Late?":bool, →"RT Loop Duration":i64)  [unwired: 1 in]
    n120 = shared-variable ".\\SharedVars.lvlib\\FromFileVelFS_rpm"() -> (w233:dbl)  [unwired: 1 in, 1 out]
    n121 = shared-variable ".\\SharedVars.lvlib\\GeneratorOn"() -> (w235:bool)  [unwired: 1 in, 1 out]
    n122 = shared-variable ".\\SharedVars.lvlib\\FromFilePitchFS_deg"() -> (w232:dbl)  [unwired: 1 in, 1 out]
    n123 = To Double Precision Float(number=w289) -> (double precision float=w310:dbl)
    n124 = shared-variable ".\\SharedVars.lvlib\\PitchAxis1On"() -> (w243:bool)  [unwired: 1 in, 1 out]
    n125 = shared-variable ".\\SharedVars.lvlib\\PitchAxis2On"() -> (w244:bool)  [unwired: 1 in, 1 out]
    n126 = shared-variable ".\\SharedVars.lvlib\\PitchAxis3On"() -> (w245:bool)  [unwired: 1 in, 1 out]
    n127 = shared-variable ".\\SharedVars.lvlib\\SimulationConstants"() -> (w272:T6)  [unwired: 1 in, 1 out]
    n128 = call "ReadIO.vi"("Zero Pitch 2"="Zero Pitch 2", "Zero Pitch 3"="Zero Pitch 3", "Zero Pitch 1"="Zero Pitch 1", "error in"=w315, "ROSCO Params In"=w316, "IO Signals In"=w314, "ArrayPairs In"=w317) -> ("error out"=w305:errorcluster, "ROSCO Params Out"=w306:T9, "IO Signals Out"=w304:T8, "ArrayPairs Out"=w307:T10, "Torque RAW (V)"=→"Torque RAW (V)":dbl)
    n129 = shared-variable ".\\SharedVars.lvlib\\SimulationConstants"() -> (w279:T6)  [unwired: 1 in, 1 out]
    n130 = Multiply(x=w310, y=w309) -> (x*y=w236:dbl)
    "Time(s)" <- w236
    n131 = Multiply(x=w258, y="Max Torque (MNm)") -> (x*y=w256:dbl)
    n132 = Multiply(x="Torque mean (MNm)", y=w258) -> (x*y=w261:dbl)
    n133 = Multiply(x=w258, y="Torque sine amp (MNm)") -> (x*y=w260:dbl)
    n134 = call "AssignStatus_v2.vi"("Time (s)"=w236, "Rosco dt (s)"=w308, "LoopCount"=w289, "Wind Estimator u(t=0)"="Wind Est. u(t=0)", "error in (no error)"=w305, "ROSCO Params In"=w306, "IO Signals In"=w304, "ArrayPairs In"=w307) -> ("error out"=w298:errorcluster, "ROSCO Params Out"=w299:T9, "IO Signals Out"=w297:T8, "ArrayPairs Out"=w300:T10)
    n135 = Bundle By Name(cluster=w277, "GeneratorOn"=w235, "Generator operating mode"="Generator operating mode", "From file velocity (rpm)"=w233, "Constant velocity setpoint (rpm)"="Const. vel setpoint (rpm)", "Ramp target velocity (rpm)"="Ramp target vel (rpm)", "Ramp time (s)"="Ramp time (s)", "Sine mean (Nm)"=w261, "Sine amp (Nm)"=w260, "Max Torque (Nm)"=w256, "Sine period (s)"="Torque sine period (s)", "Torque Ctrl P-Gain"="Torque Ctrl P-Gain", "Torque Ctrl I-Gain"="Torque Ctrl I-Gain", "Velocity Ctrl P-Gain"="Velocity Ctrl P-Gain", "Velocity Ctrl I-Gain"="Velocity Ctrl I-Gain") -> (w273:T16)
    n136 = Bundle By Name(cluster=w284, "Axis 1 On"=w243, "Axis 2 On"=w244, "Axis 3 On"=w245, "Blade pitch operating mode"="Blade pitch operating mode", "P-Gain"="Pitch P-Gain", "I-Gain"="Pitch I-Gain", "Constant setpoint (deg)"="Const. setpoint (deg)", "Sine mean (deg)"="Sine mean (deg)", "Sine amp (deg)"="Sine amp (deg)", "Sine period (s)"="Sine period (s)", "Pitch from File (deg)"=w232) -> (w282:T15)
    n137 = shared-variable ".\\SharedVars.lvlib\\CtrlLoopTime_s"(w236) -> ()  [unwired: 1 in, 1 out]
    n138 = call "CreateSwapArray_v4.vi"("Loop count"=w289, "error in (no error)"=w298, "ROSCO Params"=w299, "IO Signals In"=w297, "ArrayPairs"=w300) -> ("error out"=w293:errorcluster, "ROSCO Params Out"=w294:T9, "IO Signals Out"=w292:T8, "ArrayPairs Out"=w295:T10)  [unwired: 3 in]
    n139 = Unbundle By Name(w279) -> ("ScaleFactor"=w278:dbl)
    n140 = Unbundle By Name(w272) -> ("ScaleFactor"=w271:dbl)
    n141 = call "CallRosco_v2.vi"("StopLV"="Stop LabVIEW", "error in (no error)"=w293, "ROSCO Params in"=w294, "IO Signals In"=w292, "ArrayPairs"=w295) -> ("error out"=w290:errorcluster, "ROSCO Params Out"=w291:T9, "IO Signals Out"=w312:T8, "ArrayPairs Out"=w313:T10)  [unwired: 3 in]
    n142 = call "ScalePitchCtrl.vi"("Enum"=ScalingEnum."Full scale -> Model scale", "Scale Factor"=w278, "PitchCtrl (In)"=w282) -> ("PitchCtrl (Out)"=w281:T15)  [unwired: 8 in]
    n143 = Unbundle By Name(w313) -> ("TorqueSetpoint_Nm.Value"=w318:dbl)
    n144 = call "ScaleGenCtrl.vi"("Scale Dir"=ScalingEnum."Full scale -> Model scale", "Scale factor"=w271, "Gen Control (In)"=w273) -> ("Gen Control (Out)"=w251:T16)  [unwired: 8 in]
    n145 = Unbundle By Name(w312) -> ("pitch1Position (rad)"=w311:dbl)
    n146 = call "PitchCtrl.vi"("ArrayPairs In"=w313, "PitchCtrl"=w281, "IO Signals In"=w312, "ROSCO Params in"=w291, "error in (no error)"=w290, "Time (s)"=w236) -> ("ArrayPairs Out"=w269:T10, "IO Signals Out"=w268:T8, "ROSCO Params Out"=w267:T9, "Pitch setpoint (rad)"=w283:dbl, "error out"=w266:errorcluster)  [unwired: 5 in]
    n147 = shared-variable ".\\SharedVars.lvlib\\PitchSetpoint_rad"(w283) -> ()  [unwired: 1 in, 1 out]
    n148 = shared-variable ".\\SharedVars.lvlib\\PitchCtrl"(w281) -> ()  [unwired: 1 in, 1 out]
    n149 = shared-variable ".\\SharedVars.lvlib\\GenCtrl"(w251) -> ()  [unwired: 1 in, 1 out]
    n150 = call "GenCtrl.vi"("Loop Time (s)"=w236, "Gen Control"=w251, "error in (no error)"=w266, "ROSCO Params in"=w267, "IO Signals In"=w268, "ArrayPairs In"=w269) -> ("error out"=w263:errorcluster, "ROSCO Params Out"=w264:T9, "IO Signals Out"=w240:T8, "ArrayPairs Out"=w265:T10, "Velocity setpoint (rad/s)"=w249:dbl, "Torque setpoint (Nm)"=w250:dbl)
    "Torque setpoint (Nm)" <- w250
    n151 = shared-variable ".\\SharedVars.lvlib\\GenTorqueSetpoint_Nm"(w250) -> ()  [unwired: 1 in, 1 out]
    n152 = shared-variable ".\\SharedVars.lvlib\\GenVelocitySetpoint_radps"(w249) -> ()  [unwired: 1 in, 1 out]
    n153 = shared-variable ".\\SharedVars.lvlib\\SIM-GenTorque_Nm"(w318) -> ()  [unwired: 1 in, 1 out]
    n154 = shared-variable ".\\SharedVars.lvlib\\SIM-BladePitch_rad"(w311) -> ()  [unwired: 1 in, 1 out]
    n155 = Unbundle By Name(w240) -> ("torqueSensor (Nm)"=w239:dbl)
    n156 = shared-variable ".\\SharedVars.lvlib\\IOSignals"(w240) -> ()  [unwired: 1 in, 1 out]
    n157 = shared-variable ".\\SharedVars.lvlib\\RoscoParams"(w264) -> ()  [unwired: 1 in, 1 out]
    n158 = shared-variable ".\\SharedVars.lvlib\\RoscoPairs"(w265) -> ()  [unwired: 1 in, 1 out]
    n159 = Or(x=w263, y="Stop LabVIEW") -> (x .or. y?=w321:bool)
    n160 = call <vilib>:"Mean PtByPt.vi"("x"=w239, "sample length"=20) -> ("mean"=w237:dbl)  [unwired: 2 in, 1 out]
    n161 = shared-variable ".\\SharedVars.lvlib\\TorqueSensorMean_Nm"(w237) -> ()  [unwired: 1 in, 1 out]
    n162 = shared-variable ".\\SharedVars.lvlib\\StopLabVIEW"(w321) -> ()  [unwired: 1 in, 1 out]
    n163 = node-c288() -> ()  [unwired: 1 in, 1 out]
  }
  n164 = timed-loop {
    timing: w48 -> [_]
    timing-out: [_] -> w47
    tunnel: w39 -> [w362]
    tunnel: w38 -> [w350]
    tunnel: w37 -> [w361]
    tunnel: w23 -> [w338]
    shift-right: [w329] -> _
    shift-left: 0.5236 -> [w330]
    i -> [w355]
    stop <- w364 stop-if-true
    # "a*dt"
    # "a=1/J*(Ta-Tg)"
    # "Simulate the generator speed for now. Replace this once the actual generator speed signal is available"
    # "dt"
    # "(Ta-Tg)"
    # "Generate Simulation Signals - Can remove this code for actual operation"
    n165 = node-c288() -> (→"SimLoop Late?":bool)  [unwired: 1 in, 1 out]
    n166 = To Double Precision Float(number=w355) -> (double precision float=w354:dbl)
    n167 = shared-variable ".\\SharedVars.lvlib\\SIM-GenSpeed_rad_s"() -> (w336:dbl)  [unwired: 1 in, 1 out]
    n168 = shared-variable ".\\SharedVars.lvlib\\SIM-BladePitch_rad"() -> (w334:dbl)  [unwired: 1 in, 1 out]
    n169 = Divide(x=w354, y=1000.0) -> (x/y=w346:dbl)
    n170 = call "WindSimulator.vi"("Sine Mean (m/s)"="Sine Mean (m/s)", "Sine Amp (m/s)"="Sine Amp (m/s)", "Sine Freq (Hz)"="Sine Freq (Hz)", "Ramp Start u(m/s)"="Ramp Start u(m/s)", "Ramp End u(m/s)"="Ramp End u(m/s)", "Ramp Time (s)"="Ramp Time (s)", "Const. Amp (m/s)"="Const. Amp (m/s)", "Wind Simulation Mode"="Wind Simulation Mode", "Loop Time (s)"=w346) -> ("Wind Speed (m/s)"=w345:dbl, "Ramp time (s)"=→"Ramp time (s)":dbl)  [unwired: 9 in]
    "Wind Speed (m/s)" <- w345
    n171 = shared-variable ".\\SharedVars.lvlib\\SIM-GenTorque_Nm"() -> (w335:dbl)  [unwired: 1 in, 1 out]
    "SIM-GenTorque_Nm" <- w335
    n172 = call "RadToDeg.vi"("rad"=w334) -> ("deg"=w353:dbl)
    n173 = shared-variable ".\\SharedVars.lvlib\\SIM-WindSpeed_m_s"(w345) -> ()  [unwired: 1 in, 1 out]
    n174 = Unbundle By Name(T6 {"Ngear"=1.0, "RotorInertia"=318628128.0, "GeneratorEff"=0.9700000286102295, "RotorRadius"=120.0, "Rho"=1.225000023841858, "NumBlades"=1, "ScaleFactor"=3.0} ("SimulationConst")) -> ("RotorInertia"=w358:dbl)
    n175 = call "CalcAeroTq.vi"("GenSpeed"=w336, "WindSpeed"=w345, "Xi"=w353, "SimulationConst"=T6 {"Ngear"=1.0, "RotorInertia"=318628128.0, "GeneratorEff"=0.9700000286102295, "RotorRadius"=120.0, "Rho"=1.225000023841858, "NumBlades"=1, "ScaleFactor"=3.0}, "tsr(Y)"=w361, "pitch (X)"=w350, "Cp(Z)"=w362) -> ("Cp"=w328:dbl, "Ta"=w352:dbl)  [unwired: 2 in]
    "SIM-Cp" <- w328
    n176 = To Double Precision Float(number=w358) -> (double precision float=w356:dbl)
    n177 = Subtract(x=w352, y=w335) -> (x-y=w351:dbl)
    n178 = shared-variable ".\\SharedVars.lvlib\\SIM-Cp"(w328) -> ()  [unwired: 1 in, 1 out]
    n179 = shared-variable ".\\SharedVars.lvlib\\SIM-AeroTorque_Nm"(w352) -> ()  [unwired: 1 in, 1 out]
    n180 = Divide(x=w351, y=w356) -> (x/y=w333:dbl)
    n181 = To Double Precision Float(number=w338) -> (double precision float=w339:dbl)
    n182 = Divide(x=w339, y=1000.0) -> (x/y=w332:dbl)
    n183 = Multiply(x=w333, y=w332) -> (x*y=w331:dbl)
    n184 = Add(x=w330, y=w331) -> (x+y=w329:dbl)
    n185 = shared-variable ".\\SharedVars.lvlib\\StopLabVIEW"() -> (w364:bool)  [unwired: 1 in, 1 out]
    n186 = shared-variable ".\\SharedVars.lvlib\\SIM-GenSpeed_rad_s"(w329) -> ()  [unwired: 1 in, 1 out]
    n187 = node-c288() -> ()  [unwired: 1 in, 1 out]
  }
  n188 = timed-loop {
    timing: w35 -> [_]
    timing-out: [_] -> w34
    stop <- w387 stop-if-true
    # "Axis No. 1"
    # "State logic"
    n189 = node-c288() -> (→"State logic late?":bool)  [unwired: 1 in]
    n190 = shared-variable ".\\SharedVars.lvlib\\IOSignals"() -> (w379:T8)  [unwired: 1 in, 1 out]
    n191 = disable-structure shown="Disabled" {
      disable-tunnel: w379 -> [w407 _]
      disable-tunnel: "Clear Pitch Actuator Faults (x3)" -> [w403 _]
      disable-tunnel: "Enable Pitch Actuators (x3)" -> [w402 _]
      frame Disabled {
        # "ADD ctrl word output here once axis connected"
        # "ADD ctrl word output here once axis connected"
        # "Axis No. 3"
        # "Axis No. 2"
        n192 = call "ElmoInterface.vi"("Enable"=w402, "Clear faults"=w403, "Axis No."=u32 2, "IO Signals"=w407) -> ("Control word"=→"Pitch axis 2 ctrl word":u16, "Elmo State Cluster Out"=w405:T18)  [unwired: 6 in]
        n193 = call "ElmoInterface.vi"("Enable"=w402, "Clear faults"=w403, "Axis No."=u32 3, "IO Signals"=w407) -> ("Control word"=→"Pitch axis 3 ctrl word":u16, "Elmo State Cluster Out"=w401:T18)  [unwired: 6 in]
        n194 = Unbundle By Name(w405) -> ("Elmo State"=→"Pitch Axis 2":string, "Elmo Operational"=w392:bool, "Elmo Warning"=→"Axis 2 Warning":bool, "Elmo Fault"=→"Axis 2 Fault":bool)
        "Axis 2 Operational" <- w392
        n195 = Unbundle By Name(w401) -> ("Elmo State"=→"Pitch Axis 3":string, "Elmo Operational"=w391:bool, "Elmo Warning"=→"Axis 3 Warning":bool, "Elmo Fault"=→"Axis 3 Fault":bool)
        "Axis 3 Operational" <- w391
        n196 = shared-variable ".\\SharedVars.lvlib\\PitchAxis2On"(w392) -> ()  [unwired: 1 in, 1 out]
        n197 = shared-variable ".\\SharedVars.lvlib\\PitchAxis3On"(w391) -> ()  [unwired: 1 in, 1 out]
      }
      frame Enabled {
      }
    }
    n198 = call "AccelnetInterface.vi"("Enable"="Enable Accelnet", "Clear Faults"="Clear Accelnet Faults", "IO Signals"=w379) -> ("Control word"=w382:u16, "Accelnet State"=w386:T19)  [unwired: 7 in]
    "Gen ctrl word" <- w382
    n199 = call "ElmoInterface.vi"("Enable"="Enable Pitch Actuators (x3)", "Clear faults"="Clear Pitch Actuator Faults (x3)", "Axis No."=u32 1, "IO Signals"=w379) -> ("Control word"=w371:u16, "Elmo State Cluster Out"=w378:T18)  [unwired: 6 in]
    "Pitch axis 1 ctrl word" <- w371
    n200 = Unbundle By Name(w386) -> ("State String"=→"Main generator state":string, "Accelnet Warning"=→"Generator Warning":bool, "Accelnet Fault"=→"Generator Fault":bool, "Accelnet Operational"=w369:bool)
    "Generator Operational" <- w369
    n201 = shared-variable "NI-cRIO-9038-01A42455\\EtherCAT Master\\MainGen\\Receive PDO 7 CST-Control word"(w382) -> ()  [unwired: 1 in, 1 out]
    n202 = Unbundle By Name(w378) -> ("Elmo State"=→"Pitch Axis 1":string, "Elmo Operational"=w368:bool, "Elmo Warning"=→"Axis 1 Warning":bool, "Elmo Fault"=→"Axis 1 Fault":bool)
    "Axis 1 Operational" <- w368
    n203 = shared-variable "NI-cRIO-9038-01A42455\\EtherCAT Master\\PitchBlade1\\Outputs-Control word"(w371) -> ()  [unwired: 1 in, 1 out]
    n204 = shared-variable ".\\SharedVars.lvlib\\PitchAxis1On"(w368) -> ()  [unwired: 1 in, 1 out]
    n205 = shared-variable ".\\SharedVars.lvlib\\GeneratorOn"(w369) -> ()  [unwired: 1 in, 1 out]
    n206 = shared-variable ".\\SharedVars.lvlib\\StopLabVIEW"() -> (w387:bool)  [unwired: 1 in, 1 out]
    n207 = node-c288() -> ()  [unwired: 1 in, 1 out]
  }
  n208 = timed-loop {
    timing: w10 -> [_]
    timing-out: [_] -> w9
    tunnel: w3 -> [w412]
    tunnel: w2 -> [w416]
    tunnel: w1 -> [w411]
    stop <- w422 stop-if-true
    n209 = node-c288() -> (→"Loop duration (ms)":i64)  [unwired: 1 in]
    n210 = shared-variable ".\\SharedVars.lvlib\\SimulationConstants"() -> (w420:T6)  [unwired: 1 in, 1 out]
    n211 = shared-variable ".\\SharedVars.lvlib\\CtrlLoopTime_s"() -> (w421:dbl)  [unwired: 1 in, 1 out]
    n212 = Unbundle By Name(w420) -> ("ScaleFactor"=w419:dbl)
    n213 = call "ScaleTime.vi"("Scale Dir"=ScalingEnum."Model scale -> Full scale", "Scale factor"=w419, "Time (In)"=w421) -> ("Time OUT (Out)"=w415:dbl)  [unwired: 8 in]
    "Time FS (s)" <- w415
    n214 = Subtract(x=w416, y=w415) -> (x-y=w414:dbl[])
    n215 = Absolute Value(x=w414) -> (abs(x)=w413:dbl[])
    n216 = Array Max & Min(array=w413) -> (min index (indices)=w410:i32)  [unwired: 3 out]
    "Time index" <- w410
    n217 = Index Array(array=w412, index=w410) -> (element=w409:dbl)
    "Pitch FS (deg)" <- w409
    n218 = Index Array(array=w411, index=w410) -> (element=w408:dbl)
    "Vel FS (rpm)" <- w408
    n219 = shared-variable ".\\SharedVars.lvlib\\FromFileVelFS_rpm"(w408) -> ()  [unwired: 1 in, 1 out]
    n220 = shared-variable ".\\SharedVars.lvlib\\FromFilePitchFS_deg"(w409) -> ()  [unwired: 1 in, 1 out]
    n221 = shared-variable ".\\SharedVars.lvlib\\StopLabVIEW"() -> (w422:bool)  [unwired: 1 in, 1 out]
    n222 = node-c288() -> ()  [unwired: 1 in, 1 out]
  }
  n223 = timed-loop {
    timing: w30 -> [_]
    timing-out: [_] -> w29
    tunnel: w27 -> [w457]
    i -> [w449]
    stop <- w458 stop-if-true
    # "The sim variables are added temporarily to the file writing for comparision purposes"
    # "Data recording to RT buffer"
    n224 = node-c288() -> (→"FIFO Loop Late?":bool)  [unwired: 1 in]
    n225 = shared-variable ".\\SharedVars.lvlib\\WriteData"() -> (w450:bool)  [unwired: 1 in, 1 out]
    n226 = call "FileWriteTiming.vi"("Loop counter"=w449, "WriteData"=w450) -> ("Write counter"=w447:i32, "Time (s)"=w448:dbl)  [unwired: 8 in]
    n227 = shared-variable ".\\SharedVars.lvlib\\RoscoPairs"() -> (w432:T10)  [unwired: 1 in, 1 out]
    n228 = shared-variable ".\\SharedVars.lvlib\\IOSignals"() -> (w454:T8)  [unwired: 1 in, 1 out]
    n229 = To Double Precision Float(number=w447) -> (double precision float=w455:dbl)
    n230 = Unbundle By Name(w432) -> ("BladePitchSetpoint_rad.Value"=w431:dbl, "TorqueSetpoint_Nm.Value"=w430:dbl)
    n231 = shared-variable ".\\SharedVars.lvlib\\SIM-AeroTorque_Nm"() -> (w427:dbl)  [unwired: 1 in, 1 out]
    n232 = shared-variable ".\\SharedVars.lvlib\\SIM-WindSpeed_m_s"() -> (w429:dbl)  [unwired: 1 in, 1 out]
    n233 = shared-variable ".\\SharedVars.lvlib\\SIM-GenSpeed_rad_s"() -> (w428:dbl)  [unwired: 1 in, 1 out]
    n234 = Unbundle By Name(w454) -> ("mainGenPosition (rad)"=w453:dbl, "mainGenVelocity (rad/s)"=w452:dbl, "mainGenTorque (Nm)"=w451:dbl, "mainGenStatus"=w445:u16, "pitch1Position (rad)"=w444:dbl, "pitch1Velocity (rad/s)"=w443:dbl, "pitch1Status"=w441:u16, "pitch2Position (rad)"=w440:dbl, "pitch2Velocity (rad/s)"=w439:dbl, "pitch2Status"=w438:u16, "pitch3Position (rad)"=w436:dbl, "pitch3Velocity (rad/s)"=w435:dbl, "pitch3Status"=w434:u16)
    n235 = shared-variable ".\\SharedVars.lvlib\\SIM-Cp"() -> (w426:dbl)  [unwired: 1 in, 1 out]
    n236 = To Double Precision Float(number=w441) -> (double precision float=w442:dbl)
    n237 = To Double Precision Float(number=w438) -> (double precision float=w437:dbl)
    n238 = To Double Precision Float(number=w434) -> (double precision float=w433:dbl)
    n239 = To Double Precision Float(number=w445) -> (double precision float=w446:dbl)
    n240 = Bundle By Name(cluster=T7 {"genSpeed_rad_s"=0.0, "genTorque_Nm"=0.0, "dataLoopCounter"=0.0, "genStatus"=0.0, "pitch1Position_rad"=0.0, "pitch1Velocity_rad_s"=0.0, "pitch1Status"=0.0, "dataTime_s"=0.0, "genPosition_rad"=0.0, "pitch2Position_rad"=0.0, "pitch2Velocity_rad_s"=0.0, "pitch2Status"=0.0, "pitch3Position_rad"=0.0, "pitch3Velocity_rad_s"=0.0, "pitch3Status"=0.0, "pitchSetpoint_rad"=0.0, "torqueSetpoint_Nm"=0.0, "simUWind_m_s"=0.0, "simGenSpeed_rad_s"=0.0, "simTa_Nm"=0.0, "simCp"=0.0} ("SwapIn"), "dataTime_s"=w448, "dataLoopCounter"=w455, "genPosition_rad"=w453, "genSpeed_rad_s"=w452, "genTorque_Nm"=w451, "genStatus"=w446, "pitch1Position_rad"=w444, "pitch1Velocity_rad_s"=w443, "pitch1Status"=w442, "pitch2Position_rad"=w440, "pitch2Velocity_rad_s"=w439, "pitch2Status"=w437, "pitch3Position_rad"=w436, "pitch3Velocity_rad_s"=w435, "pitch3Status"=w433, "pitchSetpoint_rad"=w431, "torqueSetpoint_Nm"=w430, "simUWind_m_s"=w429, "simGenSpeed_rad_s"=w428, "simTa_Nm"=w427, "simCp"=w426) -> (w460:T7)
    n241 = call "FileBuffer.vi"("Write Data"=w450, "FileDataChannel"=w460, "Refnum in"=w457) -> ("dataTime_s"=→"File Write (s)":dbl, "# elements"=→"#RT FIFO":u32)  [unwired: 7 in]
    n242 = shared-variable ".\\SharedVars.lvlib\\StopLabVIEW"() -> (w458:bool)  [unwired: 1 in, 1 out]
    n243 = node-c288() -> ()  [unwired: 1 in, 1 out]
  }
  n244 = while {
    shift-right: [w469] -> _
    shift-left: _ -> [w470]
    shift-right: [w476] -> _
    shift-left: FALSE -> [w477]
    shift-right: [w479] -> w41
    shift-left: errorcluster {"status"=FALSE, "code"=0, "source"=""} ("error out") -> [w478]
    tunnel: "focalC1" -> [w472]
    tunnel: w45 -> [w473]
    tunnel: w27 -> [w474]
    stop <- w481 stop-if-true
    # "Access the file system every 200ms, writing buffered data"
    # "Create directory if doesnt exist"
    # "File access loop (non RT loop, read from RT buffer)"
    n245 = Wait (ms)(milliseconds to wait=u32 200) -> ()  [unwired: 1 out]
    n246 = call "CheckFIleWriteStatus.vi"("WriteDataButtonVal"="WriteData", "WritePrevVal"=w477, "Refnum in"=w470, "Base filename"="Base filename", "File path"=path "/home/lvuser/focal") -> ("File Name"=→"File Name":string, "Refnum out"=w469:refnum<k34>, "WriteCurrentVal"=w476:bool)  [unwired: 4 in]
    n247 = shared-variable ".\\SharedVars.lvlib\\WriteData"("WriteData") -> ()  [unwired: 1 in, 1 out]
    n248 = call "WriteToFile-v2.vi"("Refnum in"=w469, "Group Name"=w472, "Channel Names"=w473, "rt fifo"=w474, "Write?"="WriteData", "error in (no error)"=w478) -> ("Writing to file"=→"Writing":bool, "error out"=w479:errorcluster)  [unwired: 7 in, 1 out]
    n249 = shared-variable ".\\SharedVars.lvlib\\StopLabVIEW"() -> (w482:bool)  [unwired: 1 in, 1 out]
    n250 = Or(x=w479, y=w482) -> (x .or. y?=w481:bool)
  }
  n251 = node-c288(w34) -> ()  [unwired: 1 out]
  n252 = node-c288(w29) -> ()  [unwired: 1 out]
  n253 = node-c288(w9) -> ()  [unwired: 1 out]
  n254 = node-c288(w21) -> ()  [unwired: 1 out]
  n255 = node-c288(w47) -> ()  [unwired: 1 out]
  n256 = call <vilib>:"Simple Error Handler.vi"("error in (no error)"=w19) -> ()  [unwired: 4 in, 5 out]
  n257 = call <vilib>:"Simple Error Handler.vi"("error in (no error)"=w41) -> ()  [unwired: 4 in, 5 out]
  "MS Pitch Blade 2 (deg)" <- 0.0 ("MS Pitch Blade 2 (deg)")
  "MS Pitch Blade 3 (deg)" <- 0.0 ("MS Pitch Blade 3 (deg)")
  "Setpoints" <- w4
